vi "GDI Resize Image.vi"(4 "Set Background Color (T)":bool=TRUE, 5 "Background Color":u32(colorbox)=16777215, 7 "Image Data":T1, 8 "error in (no error)":errorcluster, 9 "Height":i32=400, 10 "Width":i32=800, 11 "Path":path) -> (0 "error out":errorcluster, 3 "Resized image data":T1)   [LabVIEW 2015]
doc: "Use the Windows GDI functions to resize an image. Pass in the image as the <b>Path</b> or <b>Image Data</b>. Enter also the desired <b>Width</b> and <b>Height</b>. If the image has an alpha layer the <b>Background Color</b> selected will be used.\n\n-------------\nDeveloped by Brian Hoover (hooovahh)"
uses:
  <vilib>/picture/picture.llb/imagedata.ctl
  System.Drawing
  <vilib>/wsapi/NI_WebServices.lvlib
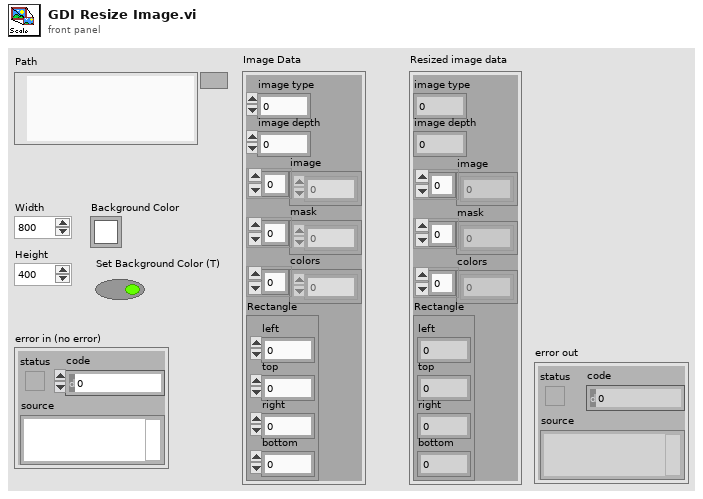
[diagram p1: front panel]
types:
  T1 = typedef "imagedata.ctl" = cluster{"image type":i32, "image depth":i32, "image":u8[], "mask":u8[], "colors":u32[], "Rectangle":cluster{"left":i16, "top":i16, "right":i16, "bottom":i16}}
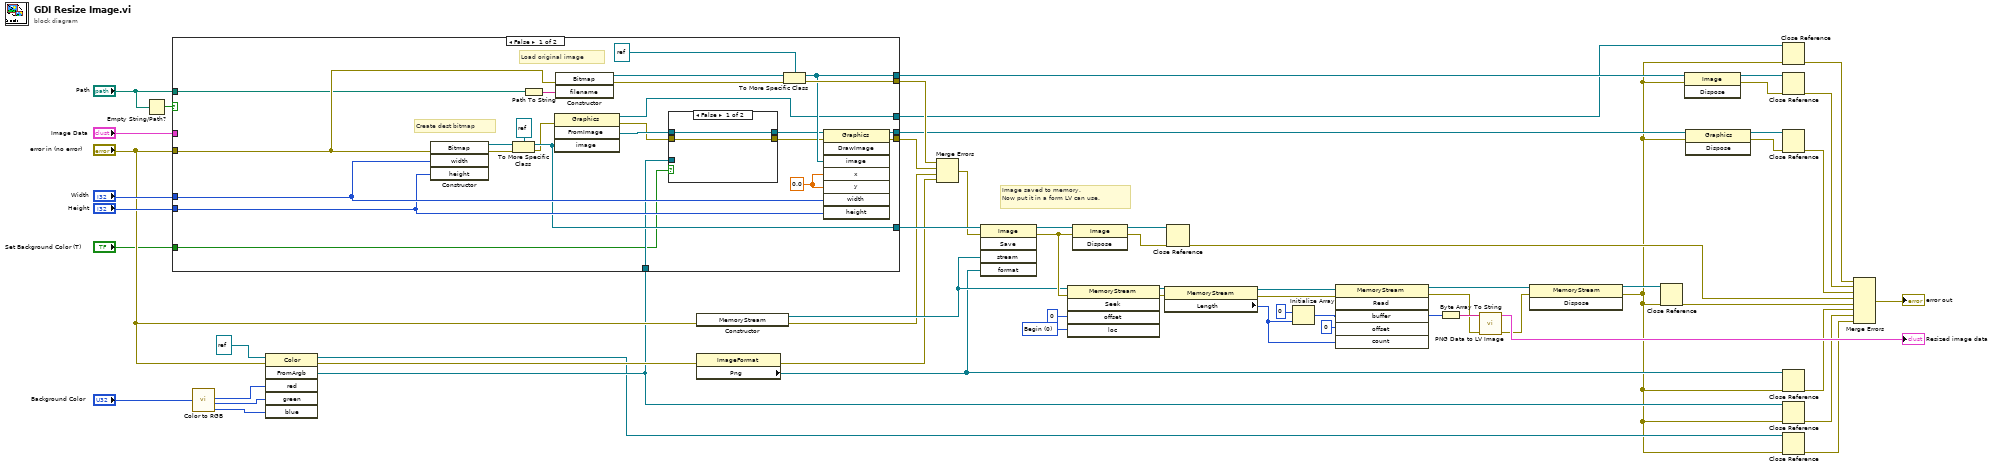
[diagram p0: block diagram]
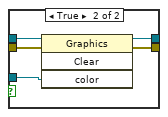
[diagram p2: hidden frame]
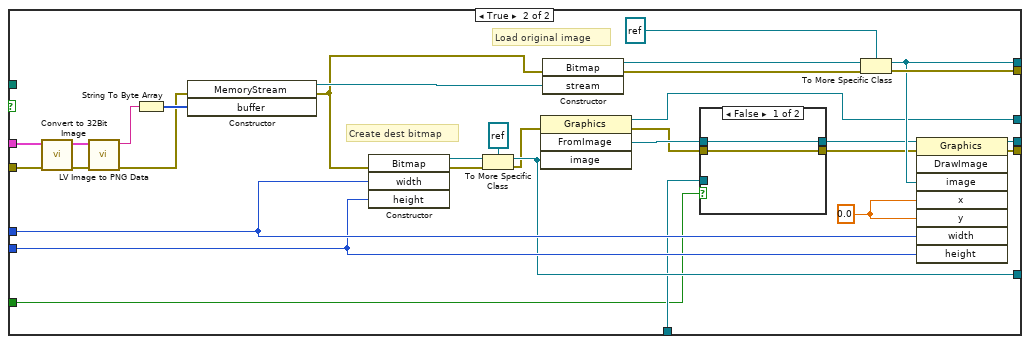
[diagram p3: hidden frame]
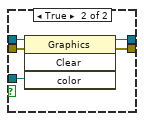
[diagram p4: hidden frame]
diagram:
  w55 = 0 items=["Begin", "Current", "End"] ("loc")
  # "Image saved to memory. \nNow put it in a form LV can use."
  n1 = Empty String/Path?(string/path="Path") -> (empty?=w17:bool)
  n2 = call <vilib>:"Color to RGB.vi"("Color"="Background Color") -> ("R"=w14:u8, "G"=w13:u8, "B"=w12:u8)  [unwired: 1 out]
  n3 = invoke class="Color" method="FromArgb"(reference=refnum<k24> refnum ("color"), error in="error in (no error)", "red"=w14, "green"=w13, "blue"=w12) -> (reference out=w7:refnum<k24>, error out=w9:errorcluster, "FromArgb"=w8:refnum<k24>)  [unwired: 1 in, 3 out]
  n4 = case shown="False" w17 {
    tunnel: "Width" -> [w83 w121]
    tunnel: "Height" -> [w82 w120]
    tunnel: [w81 w119] -> w45
    tunnel: [w78 w116] -> w43
    tunnel: [w73 w112] -> w41
    tunnel: [w72 w111] -> w40
    tunnel: [w71 w110] -> w35
    tunnel: "error in (no error)" -> [w70 w105]
    tunnel: "Path" -> [w69 _]
    tunnel: "Image Data" -> [_ w104]
    tunnel: w8 -> [w64 w96]
    tunnel: [w63 w95] -> w4
    tunnel: "Set Background Color (T)" -> [w62 w94]
    frame False {
      w86 = sgl 0.0 ("x")
      # "Create dest bitmap"
      # "Load original image"
      n5 = constructor class="Bitmap"(error in=w70, "width"=w83, "height"=w82) -> (reference out=w84:refnum<k24>, error out=w80:errorcluster)  [unwired: 2 in, 3 out]
      n6 = To More Specific Class(target class=refnum<k24> refnum, reference=w84, error in=w80) -> (specific class reference=w81:refnum<k24>, error out=w79:errorcluster)
      n7 = Path To String(path=w69) -> (string=w77:string)
      n8 = invoke class="Graphics" method="FromImage"(error in=w79, "image"=w81) -> (reference out=w63:refnum<k24>, error out=w67:errorcluster, "FromImage"=w68:refnum<k24>)  [unwired: 2 in, 1 out]
      n9 = constructor class="Bitmap"(error in=w70, "filename"=w77) -> (reference out=w75:refnum<k24>, error out=w74:errorcluster)  [unwired: 2 in, 2 out]
      n10 = case shown="False" w62 {
        tunnel: w68 -> [w88 w93]
        tunnel: w67 -> [w87 w92]
        tunnel: [w88 w91] -> w66
        tunnel: [w87 w90] -> w65
        tunnel: w64 -> [_ w89]
        frame False {
        }
        frame True {
          n11 = invoke class="Graphics" method="Clear"(reference=w93, error in=w92, "color"=w89) -> (reference out=w91:refnum<k24>, error out=w90:errorcluster)  [unwired: 1 in, 2 out]
        }
      }
      n12 = To More Specific Class(target class=refnum<k24> refnum, reference=w75, error in=w74) -> (specific class reference=w72:refnum<k24>, error out=w73:errorcluster)
      n13 = invoke class="Graphics" method="DrawImage"(reference=w66, error in=w65, "image"=w72, "x"=w86, "y"=w86, "width"=w83, "height"=w82) -> (reference out=w71:refnum<k24>, error out=w78:errorcluster)  [unwired: 1 in, 6 out]
    }
    frame True {
      w124 = sgl 0.0 ("x")
      # "Create dest bitmap"
      # "Load original image"
      n14 = call "Convert to 32Bit Image.vi"("error in (no error)"=w105, "Image Data"=w104) -> ("error out"=w109:errorcluster, "32Bit Image Data Out"=w108:T1)  [unwired: 8 in]
      n15 = call <vilib>:"LV Image to PNG Data.vi"("error in (no error)"=w109, "image data"=w108) -> ("error out"=w101:errorcluster, "png data"=w107:string)  [unwired: 8 in]
      n16 = String To Byte Array(string=w107) -> (unsigned byte array=w106:u8[])
      n17 = constructor class="MemoryStream"(error in=w101, "buffer"=w106) -> (reference out=w103:refnum<k24>, error out=w102:errorcluster)  [unwired: 2 in, 2 out]
      n18 = constructor class="Bitmap"(error in=w102, "width"=w121, "height"=w120) -> (reference out=w122:refnum<k24>, error out=w118:errorcluster)  [unwired: 2 in, 3 out]
      n19 = To More Specific Class(target class=refnum<k24> refnum, reference=w122, error in=w118) -> (specific class reference=w119:refnum<k24>, error out=w117:errorcluster)
      n20 = invoke class="Graphics" method="FromImage"(error in=w117, "image"=w119) -> (reference out=w95:refnum<k24>, error out=w99:errorcluster, "FromImage"=w100:refnum<k24>)  [unwired: 2 in, 1 out]
      n21 = constructor class="Bitmap"(error in=w102, "stream"=w103) -> (reference out=w114:refnum<k24>, error out=w113:errorcluster)  [unwired: 2 in, 2 out]
      n22 = case shown="False" w94 {
        tunnel: w100 -> [w126 w131]
        tunnel: w99 -> [w125 w130]
        tunnel: [w125 w129] -> w98
        tunnel: [w126 w128] -> w97
        tunnel: w96 -> [_ w127]
        frame False {
        }
        frame True {
          n23 = invoke class="Graphics" method="Clear"(reference=w131, error in=w130, "color"=w127) -> (reference out=w128:refnum<k24>, error out=w129:errorcluster)  [unwired: 1 in, 2 out]
        }
      }
      n24 = To More Specific Class(target class=refnum<k24> refnum, reference=w114, error in=w113) -> (specific class reference=w111:refnum<k24>, error out=w112:errorcluster)
      n25 = invoke class="Graphics" method="DrawImage"(reference=w97, error in=w98, "image"=w111, "x"=w124, "y"=w124, "width"=w121, "height"=w120) -> (reference out=w110:refnum<k24>, error out=w116:errorcluster)  [unwired: 1 in, 6 out]
    }
  }
  n26 = constructor class="MemoryStream"(error in="error in (no error)") -> (reference out=w42:refnum<k24>, error out=w26:errorcluster)  [unwired: 2 in, 1 out]
  n27 = property class="ImageFormat"(error in=w9) -> (error out=w25:errorcluster, "Png"=w33:refnum<k24>)  [unwired: 1 in, 1 out]
  n28 = Merge Errors(w41, w43, w26, w25) -> (w36:errorcluster)
  n29 = invoke class="Image" method="Save"(reference=w45, error in=w36, "stream"=w42, "format"=w33) -> (reference out=w59:refnum<k24>, error out=w47:errorcluster)  [unwired: 1 in, 3 out]
  n30 = invoke class="MemoryStream" method="Seek"(reference=w42, error in=w47, "offset"=i64 0, "loc"=w55) -> (reference out=w58:refnum<k24>, error out=w57:errorcluster)  [unwired: 1 in, 3 out]
  n31 = invoke class="Image" method="Dispose"(reference=w59, error in=w47) -> (reference out=w37:refnum<k24>, error out=w31:errorcluster)  [unwired: 1 in, 1 out]
  n32 = property class="MemoryStream"(reference=w58, error in=w57) -> (reference out=w53:refnum<k24>, error out=w52:errorcluster, "Length"=w50:i64)
  n33 = Close Reference(reference=w37, error in (no error)=w31) -> (error out=w28:errorcluster)
  n34 = Initialize Array(u8 0 ("element"), w50) -> (w51:u8[])
  n35 = invoke class="MemoryStream" method="Read"(reference=w53, error in=w52, "buffer"=w51, "offset"=0, "count"=w50) -> (reference out=w48:refnum<k24>, error out=w30:errorcluster, "buffer"=w46:u8[])  [unwired: 1 in, 3 out]
  n36 = Byte Array To String(unsigned byte array=w46) -> (string=w44:string)
  n37 = call <vilib>:"PNG Data to LV Image.vi"("error in (no error)"=w30, "png data"=w44) -> ("error out"=w29:errorcluster, "image data"=→"Resized image data":T1)  [unwired: 8 in]
  n38 = invoke class="MemoryStream" method="Dispose"(reference=w48, error in=w29) -> (reference out=w39:refnum<k24>, error out=w3:errorcluster)  [unwired: 1 in, 1 out]
  n39 = Close Reference(reference=w39, error in (no error)=w3) -> (error out=w27:errorcluster)
  n40 = invoke on="Release the file lock" class="Image" method="Dispose"(reference=w40, error in=w3) -> (reference out=w38:refnum<k24>, error out=w23:errorcluster)  [unwired: 1 in, 1 out]
  n41 = invoke class="Graphics" method="Dispose"(reference=w35, error in=w3) -> (reference out=w34:refnum<k24>, error out=w24:errorcluster)  [unwired: 1 in, 1 out]
  n42 = Close Reference(reference=w4, error in (no error)=w3) -> (error out=w2:errorcluster)
  n43 = Close Reference(reference=w38, error in (no error)=w23) -> (error out=w20:errorcluster)
  n44 = Close Reference(reference=w34, error in (no error)=w24) -> (error out=w21:errorcluster)
  n45 = Close Reference(reference=w33, error in (no error)=w3) -> (error out=w22:errorcluster)
  n46 = Close Reference(reference=w8, error in (no error)=w3) -> (error out=w6:errorcluster)
  n47 = Close Reference(reference=w7, error in (no error)=w3) -> (error out=w5:errorcluster)
  n48 = Merge Errors(w2, w20, w21, w28, w27, w22, w6, w5) -> (→"error out":errorcluster)
